vi "set array elements (dbl 1d).vi"(0 "array in":dbl[](array[numeric]), 5 "start":i32, 7 "end":i32=-1, 9 "start 2":i32, 11 "end 2":i32=-1, 12 "val":dbl) -> (4 "array out":dbl[](array[numeric]))   [LabVIEW 2012, in "common.lvlib"]
uses:
  common.lvlib
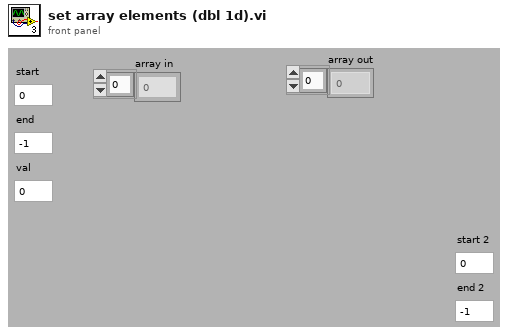
[diagram p1: front panel]
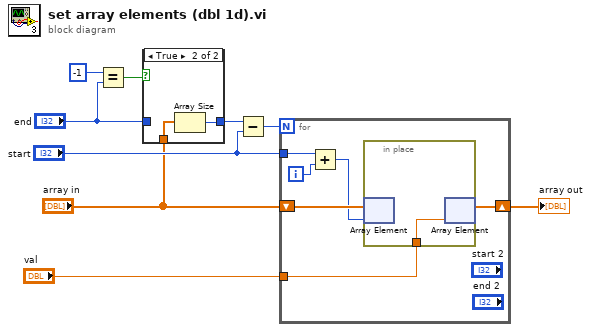
[diagram p0: block diagram]
diagram:
  n1 = Equal?(x=-1, y="end") -> (x = y?=w4:bool)
  n2 = case shown="True" w4 {
    tunnel: "end" -> [w10 _]
    tunnel: [w10 w12] -> w2
    tunnel: "array in" -> [_ w11]
    frame False {
    }
    frame True {
      n3 = Array Size(array=w11) -> (size(s)=w12:i32)
    }
  }
  n4 = Subtract(x=w2, y="start") -> (x-y=w9:i32)
  n5 = for {
    N: w9 -> [_]
    tunnel: "start" -> [w18]
    shift-right: [w13] -> w6
    shift-left: "array in" -> [w16]
    tunnel: "val" -> [w14]
    i -> [w17]
    n6 = Add(x=w18, y=w17) -> (x+y=w15:i32)
    n7 = in-place {
      in-place-border: w14 -> [w19]
      n8 = in-place-array #1(w16, w15) -> ()  [unwired: 1 out]
      n9 = in-place-array #1(w19) -> (w13:dbl[])  [unwired: 1 out]
    }
  }
  "array out" <- w6
